vi "PUERTOS ANALOG.vi"(0 "VISA \nresource\nname":refnum<visa-resource-name>, 5 "PUERTO":u8(ring) items=["PUERTOA", "PUERTOE", "PUERTOB"], 7 "CANAL":u8(ring) items=["CAD_CH0_PA_pin2", "CAD_CH1_PA_pin3", "CAD_CH2_PA_pin4", "CAD_CH3_PA_pin5", "CAD_CH4_PA_pin7", "CAD_CH5_PE_pin8", "CAD_CH6_PE_pin9", "CAD_CH7_PE_pin10", "CAD_CH8_PB_pin35", "CAD_CH9_PB_pin36", "CAD_CH10_PB_pin34", "CAD_CH11_PB_pin37", "CAD_CH12_PB_pin33"], 9 "REFERENCIA":u8(ring) items=["VDD, VSS", "Vref+", "Vref-", "Vref+, Vref-"], 11 "error":errorcluster, 12 "HABILITA":bool) -> (4 "VISA \nresource \nname":refnum<visa-resource-name>, 6 "RESULTADO":string, 8 "RESULTADO U16":u16, 15 "error":errorcluster)   [LabVIEW 2009]
panel:
  out "RESULTADO U8 2":u16
  out "RESULTADO U8":u16
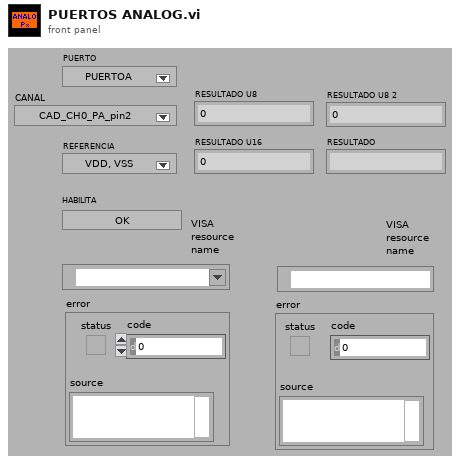
[diagram p1: front panel]
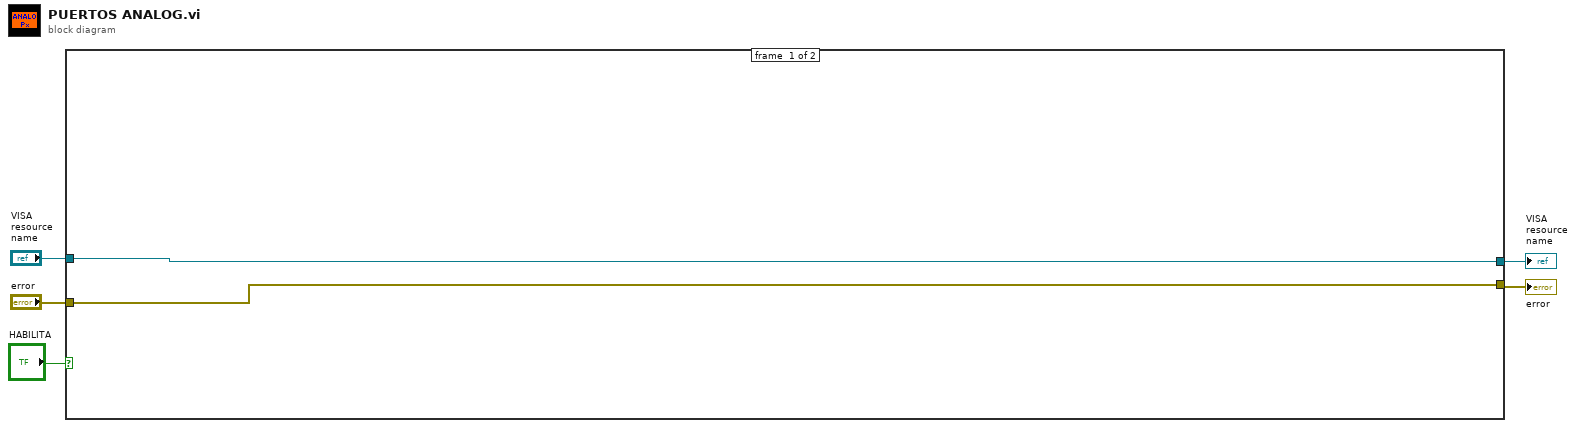
[diagram p0: block diagram]
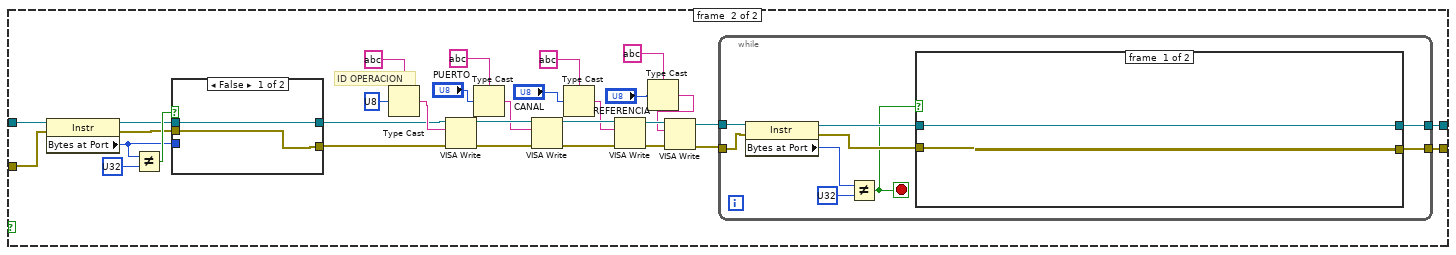
[diagram p2: hidden frame]
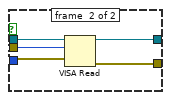
[diagram p3: hidden frame]
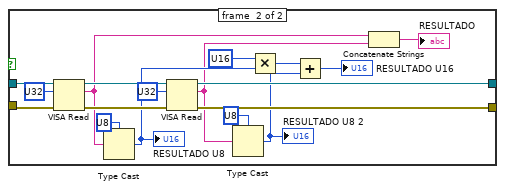
[diagram p4: hidden frame]
diagram:
  n1 = case shown="True" "HABILITA" {
    tunnel: "VISA \nresource\nname" -> [w7 w25]
    tunnel: "error" -> [w6 w24]
    tunnel: [w7 w23] -> w3
    tunnel: [w6 w22] -> w2
    frame #0 {
    }
    frame #1 {
      # "ID OPERACION"
      n2 = property class="Instr"(reference=w25, error in=w24) -> (reference out=w26:refnum<visa-resource-name>, error out=w27:errorcluster, "Bytes at Port"=w28:u32)
      n3 = Not Equal?(x=w28, y=u32 ?) -> (x != y?=w30:bool)
      n4 = case shown="False" w30 {
        tunnel: w26 -> [w40 w45]
        tunnel: w27 -> [w39 w44]
        tunnel: w28 -> [_ w43]
        tunnel: [w40 w42] -> w8
        tunnel: [w39 w41] -> w9
        frame #0 {
        }
        frame #1 {
          n5 = VISA Read(VISA resource name=w45, byte count=w43, error in (no error)=w44) -> (VISA resource name out=w42:refnum<visa-resource-name>, error out=w41:errorcluster)  [unwired: 2 out]
        }
      }
      n6 = Type Cast(type=string ?, x=u8 ?) -> (*(type *) &x=w15:string)
      n7 = VISA Write(VISA resource name=w8, write buffer=w15, error in (no error)=w9) -> (VISA resource name out=w18:refnum<visa-resource-name>, error out=w16:errorcluster)  [unwired: 1 out]
      n8 = Type Cast(type=string ?, x="PUERTO") -> (*(type *) &x=w14:string)
      n9 = VISA Write(VISA resource name=w18, write buffer=w14, error in (no error)=w16) -> (VISA resource name out=w21:refnum<visa-resource-name>, error out=w17:errorcluster)  [unwired: 1 out]
      n10 = Type Cast(type=string ?, x="CANAL") -> (*(type *) &x=w13:string)
      n11 = VISA Write(VISA resource name=w21, write buffer=w13, error in (no error)=w17) -> (VISA resource name out=w20:refnum<visa-resource-name>, error out=w19:errorcluster)  [unwired: 1 out]
      n12 = Type Cast(type=string ?, x="REFERENCIA") -> (*(type *) &x=w12:string)
      n13 = VISA Write(VISA resource name=w20, write buffer=w12, error in (no error)=w19) -> (VISA resource name out=w11:refnum<visa-resource-name>, error out=w10:errorcluster)  [unwired: 1 out]
      n14 = while {
        tunnel: [w54] -> w23
        tunnel: [w53] -> w22
        tunnel: w11 -> [w47]
        tunnel: w10 -> [w46]
        stop <- w49 stop-if-true
        n15 = property class="Instr"(reference=w47, error in=w46) -> (reference out=w52:refnum<visa-resource-name>, error out=w51:errorcluster, "Bytes at Port"=w48:u32)
        n16 = Not Equal?(x=w48, y=u32 ?) -> (x != y?=w49:bool)
        n17 = case shown="True" w49 {
          tunnel: [w56 w70] -> w54
          tunnel: [w55 w68] -> w53
          tunnel: w52 -> [w56 w72]
          tunnel: w51 -> [w55 w71]
          frame #0 {
          }
          frame #1 {
            n18 = VISA Read(VISA resource name=w72, byte count=u32 ?, error in (no error)=w71) -> (VISA resource name out=w70:refnum<visa-resource-name>, read buffer=w58:string, error out=w69:errorcluster)  [unwired: 1 out]
            n19 = Type Cast(type=u8 ?, x=w58) -> (*(type *) &x=w64:u8)
            "RESULTADO U8" <- w64
            n20 = VISA Read(VISA resource name=w70, byte count=u32 ?, error in (no error)=w69) -> (read buffer=w57:string, error out=w68:errorcluster)  [unwired: 2 out]
            n21 = Type Cast(type=u8 ?, x=w57) -> (*(type *) &x=w66:u8)
            "RESULTADO U8 2" <- w66
            n22 = Multiply(x=u16 ?, y=w64) -> (x*y=w65:u16)
            n23 = Add(x=w65, y=w66) -> (x+y=→"RESULTADO U16":u16)
            n24 = Concatenate Strings(w58, w57) -> (→"RESULTADO":string)
          }
        }
      }
    }
  }
  "VISA \nresource \nname" <- w3
  "error" <- w2
